vi "proc.util.enumToStrStepVar.vi"(10 "Step var":T1=enum."stepSetpoint") -> (2 "String":string)   [LabVIEW 2024]
uses:
  controls/typeStepVarients.ctl
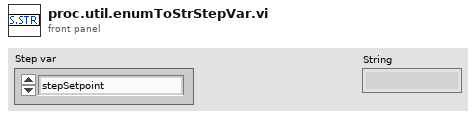
[diagram p1: front panel]
types:
  T1 = typedef "typeStepVarients.ctl" = enum16{"stepNameID", "stepFunction", "stepReport", "stepSetpoint", "stepPointer", "stepProcPointer", "stepIoPointer", "stepIoValue", "stepFilePointer", "stepMessage", "stepTimeString", "stepNumReg", "stepStrReg", "stepSeconds", "stepUnitDoseParams", "stepUnitIndex"}
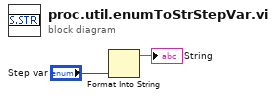
[diagram p0: block diagram]
diagram:
  n1 = Format Into String("Step var") -> (resulting string=→"String":string)  [unwired: 3 in, 1 out]
